vi "QD test types.vi"() -> ()   [LabVIEW 2018]
uses:
  Value_class/Value.lvclass
  RefferenceA/RefferenceA.lvclass
  RefferenceA2/RefferenceA2.lvclass
  <vilib>/ErrorRing/Error Ring.xnode
panel:
  out "Numeric 7":sgl
  out "Numeric 6":u16
  out "Numeric 5":i32
  out "Enum":enum16{"1", "2", "3", "4", "5"}(ring)
  out "Numeric 4":dbl
  out "Class Array":refnum<class "RefferenceA.lvclass">[](array[class])
  out "Numeric Array":i32[](array[numeric])
  out "String Array":string[](array[string])
  out "RefferenceA2":refnum<class "RefferenceA2.lvclass">
  out "Refference":refnum<class "RefferenceA.lvclass">
  out "Numeric 3":cdb
  out "Cluster":T1
  out "error constant":errorcluster
  out "Value":refnum<class "Value.lvclass">
  out "File Path":path
  out "Numeric 2":i32
  out "Numeric":dbl
  out "Time Stamp":timestamp
  out "error out 3":errorcluster
  out "Boolean":bool
  out "error out 2":errorcluster
  out "error out":errorcluster
  out "String":string
  # "This is a test VI for the data wire types"
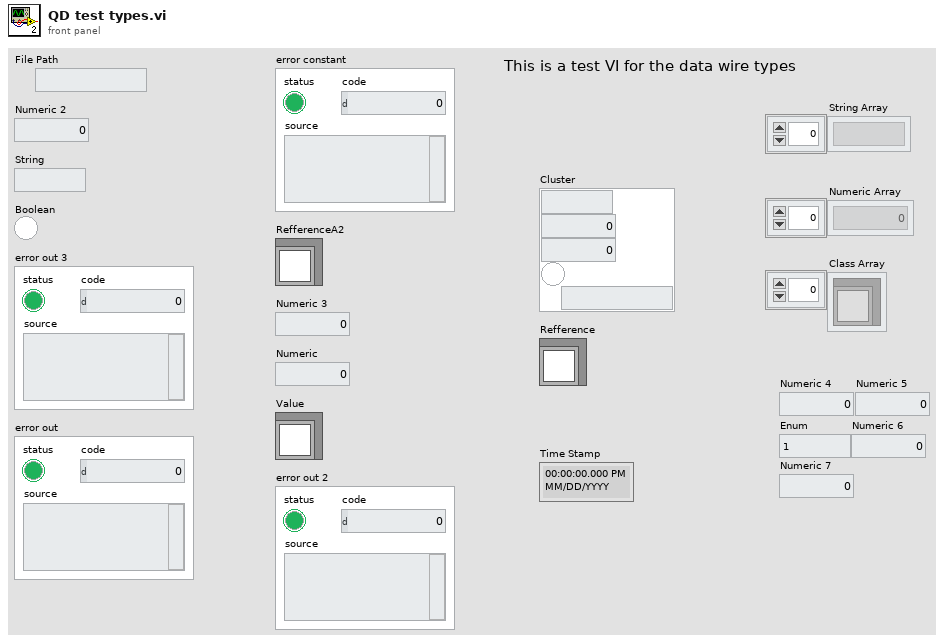
[diagram p1: front panel]
types:
  T1 = cluster{"String":string, "Numeric":i32, "Numeric":dbl, "Boolean":bool, "File Path":path}
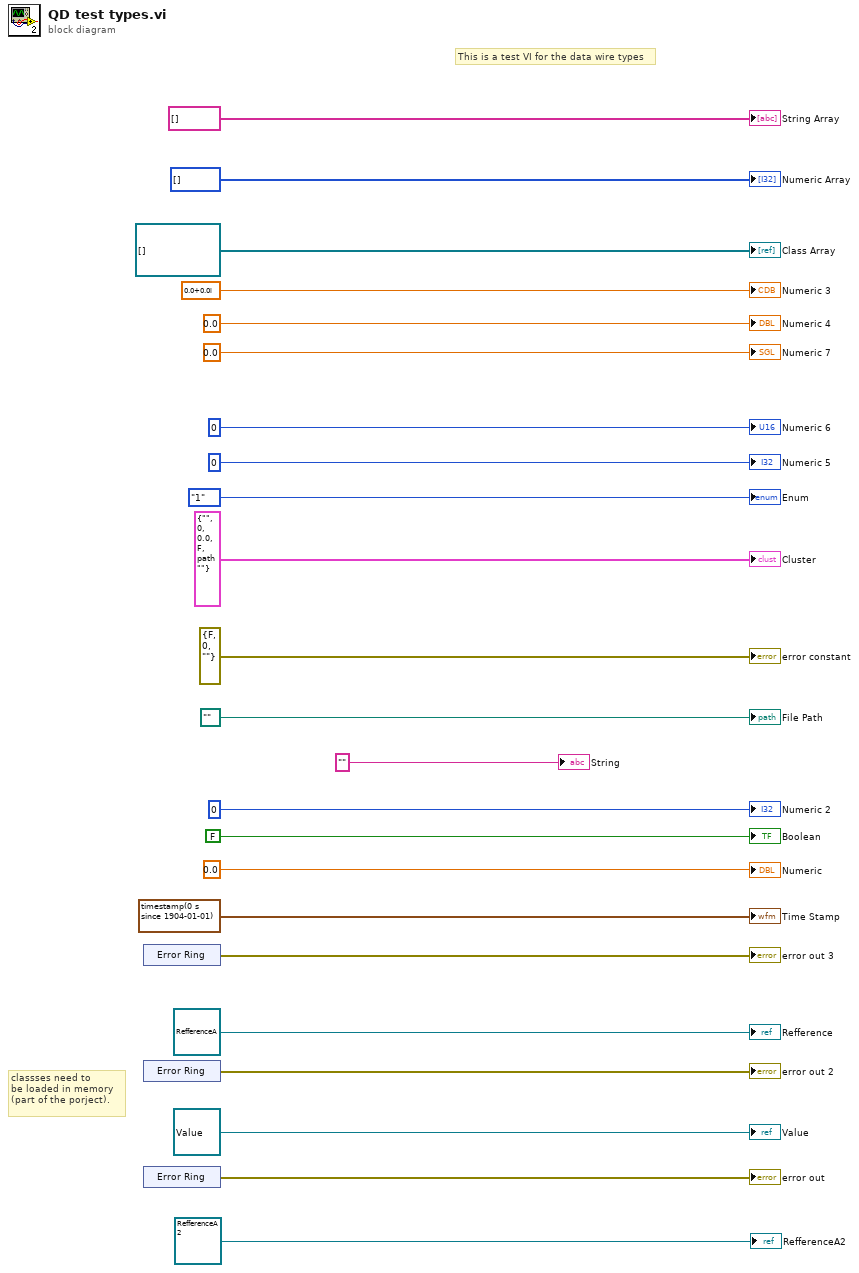
[diagram p0: block diagram]
diagram:
  # "This is a test VI for the data wire types"
  # "classses need to\nbe loaded in memory\n(part of the porject)."
  n1 = xnode ("Error Ring")() -> ("error out"=→"error out 3":errorcluster)
  n2 = xnode ("Error Ring")() -> ("error out"=→"error out 2":errorcluster)
  n3 = xnode ("Error Ring")() -> ("error out"=→"error out":errorcluster)
  "String" <- ""
  "Boolean" <- FALSE
  "Time Stamp" <- timestamp(0 s since 1904-01-01)
  "Numeric" <- sgl 0.0
  "Numeric 2" <- 0
  "File Path" <- path ""
  "Value" <- refnum<class "Value.lvclass"> refnum ("Value")
  "error constant" <- errorcluster {"status"=FALSE, "code"=0, "source"=""} ("error constant")
  "Cluster" <- cluster{string, i32, dbl, bool, path} {"", 0, 0.0, FALSE, path ""}
  "Numeric 3" <- cdb 0.0+0.0i
  "Refference" <- refnum<class "RefferenceA.lvclass"> refnum ("Refference")
  "RefferenceA2" <- refnum<class "RefferenceA2.lvclass"> refnum ("RefferenceA2")
  "String Array" <- string[] []
  "Numeric Array" <- i32[] []
  "Class Array" <- refnum<class "RefferenceA.lvclass">[] []
  "Numeric 4" <- 0.0
  "Enum" <- enum16{"1", "2", "3", "4", "5"}."1"
  "Numeric 5" <- 0
  "Numeric 6" <- u16 0
  "Numeric 7" <- sgl 0.0
